vi "SubConfocal_SetFWSpeed.vi"(7 "Confocal scanner":T1={"SDC shutter"=FALSE, "Filter wheel"=3, "FW speed"=3, "Disk spinning"=FALSE, "Disk speed (rpm)"=3000.0} {"Disk speed (rpm)" min=1500.0 max=10000.0; "FW speed" min=1 max=5 step=1; "Filter wheel" items=["CFP"=1, "GFP"=2, "mCherry"=3, "Alexa-647"=4, "OFP"=5, "empty"=6]}, 8 "Error In":errorcluster, 11 "Confocal line  (VISA IN)":refnum<visa-resource-name>="COM1") -> (0 "Error out":errorcluster, 3 "VISA OUT":refnum<visa-resource-name>)   [LabVIEW 2015]
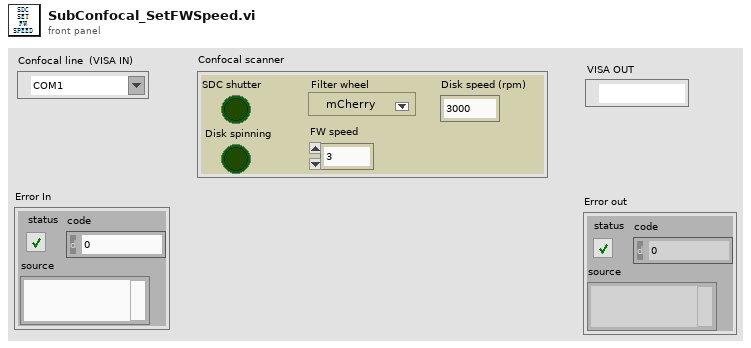
[diagram p1: front panel]
types:
  T1 = cluster{"SDC shutter":bool, "Filter wheel":u16, "FW speed":i32, "Disk spinning":bool, "Disk speed (rpm)":dbl}
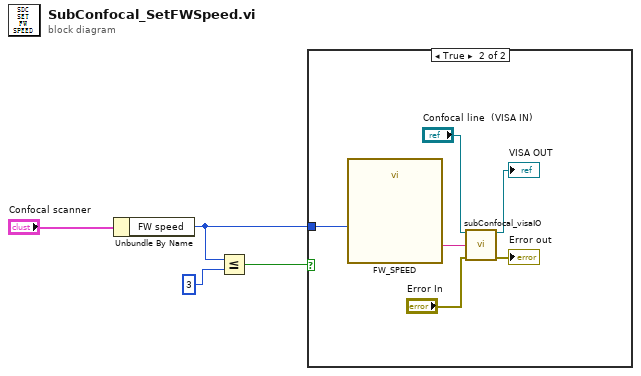
[diagram p0: block diagram]
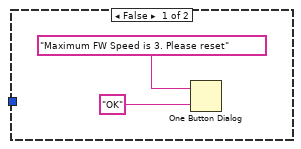
[diagram p2: hidden frame]
diagram:
  n1 = Unbundle By Name("Confocal scanner") -> ("FW speed"=w2:i32)
  n2 = Less Or Equal?(x=w2, y=3) -> (x <= y?=w1:bool)
  n3 = case shown="True" w1 {
    tunnel: w2 -> [_ w7]
    frame False {
      n4 = One Button Dialog(message="Maximum FW Speed is 3. Please reset", button name ("OK")="OK") -> ()  [unwired: 1 out]
    }
    frame True {
      n5 = call "FW_SPEED"("speed"=w7) -> ("Result"=w12:string)  [unwired: 13 in, 1 out]
      n6 = call "subConfocal_visaIO.vi"("VISA  IN"="Confocal line  (VISA IN)", "Command (to ctlr)"=w12, "error in"="Error In") -> ("VISA OUT"=→"VISA OUT":refnum<visa-resource-name>, "error out"=→"Error out":errorcluster)  [unwired: 8 in, 3 out]
    }
  }
